vi "sub_LogData_save2.vi"(8 "error in":errorcluster, 11 "Q_data":T1) -> (0 "error out":errorcluster)   [LabVIEW 2016]
uses:
  ctl/q_data.ctl
  ctl/file_path-cmd.ctl
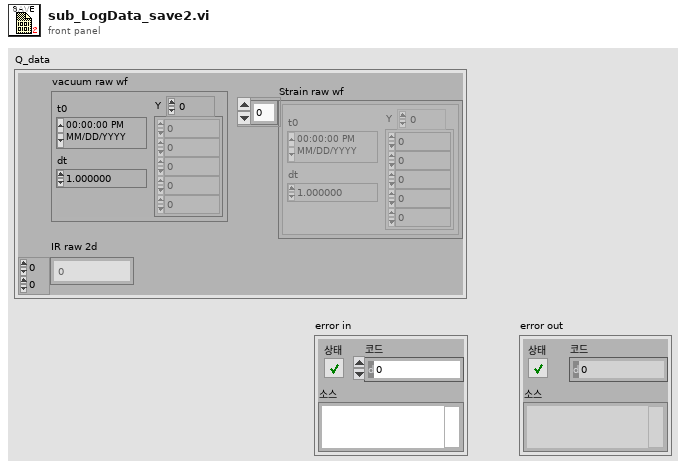
[diagram p1: front panel]
types:
  T1 = typedef "q_data.ctl" = cluster{"Strain raw wf":waveform(dbl)[], "vacuum raw wf":waveform(dbl), "IR raw 2d":i16[][]}
  T2 = typedef "file_path-cmd.ctl" = enum16{"default", "write"}
  T3 = enum16{"open", "replace", "create", "open or create", "replace or create", "replace or create with confirmation"}
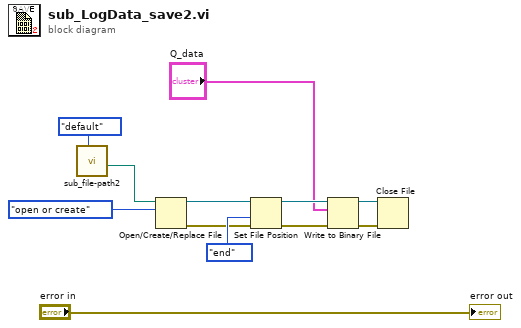
[diagram p0: block diagram]
diagram:
  n1 = call "sub_file-path2.vi"("cmd"=file_path-cmd."default") -> ("Raw log file path"=w12:path)  [unwired: 8 in, 2 out]
  n2 = Open/Create/Replace File(file path (use dialog)=w12, operation (0:open)=T3."open or create" ("동작(0:open)")) -> (refnum out=w7:refnum<file>, error out=w6:errorcluster)  [unwired: 4 in, 1 out]
  n3 = Set File Position(refnum=w7, from (0:start)=enum16{"start", "end", "current"}."end" ("시작(0:시작)"), error in=w6) -> (refnum out=w8:refnum<file>, error out=w9:errorcluster)  [unwired: 1 in]
  n4 = Write to Binary File(file (use dialog)=w8, data="Q_data", error in=w9) -> (refnum out=w5:refnum<file>, error out=w4:errorcluster)  [unwired: 3 in, 1 out]
  n5 = Close File(refnum=w5, error in=w4) -> ()  [unwired: 2 out]
  "error out" <- "error in"
